vi "Test Base64 Encoder and Decoder.vi"() -> ()   [LabVIEW 2013]
uses:
  source-base64/Serializer.Base64.lvclass/Serializer.Base64.ctl
  source-base64/Base64url_CharSet.vi
  source-base64/Write charset.vi
  source-base64/Base64_CharSet.vi
  source-base64/Encode.vi
  source-base64/Serializer.Base64.lvclass
  <vilib>/LabVIEW Open Source Project/OpenSerializer/Serializer/Serializer.lvclass
panel:
  out "Decoded String":string
  out "Encoded String":string
  out "Variant 4":variant
  out "invalid type":errorcluster
  out "error out":errorcluster
  out "Variant 2":variant
  out "Variant":variant
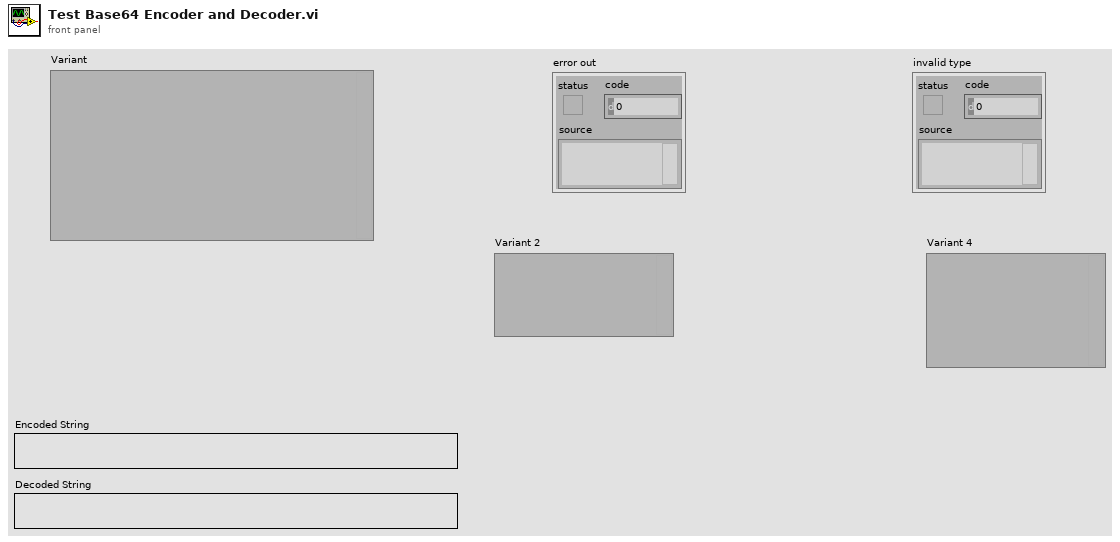
[diagram p1: front panel]
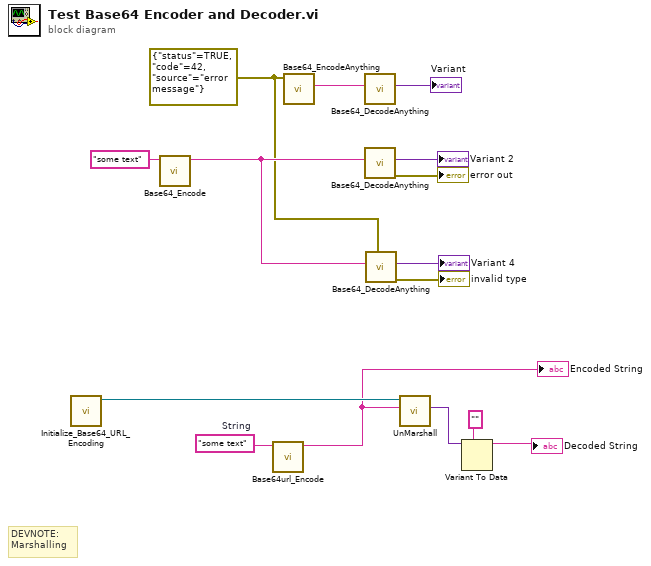
[diagram p0: block diagram]
diagram:
  w6 = "some text"  # String
  w7 = errorcluster {"status"=TRUE, "code"=42, "source"="error message"} ("error constant")
  # "DEVNOTE: \nMarshalling"
  n1 = call "Initialize_Base64_URL_Encoding.vi"() -> ("Base64 URL Encoding"=w5:refnum<class "Serializer.Base64.lvclass">)  [unwired: 11 in]
  n2 = call "Base64_Encode.vi"("String"="some text") -> ("Encoded String"=w8:string)  [unwired: 9 in, 1 out]
  n3 = call "Base64url_Encode.vi"("String"=w6) -> ("Encoded String"=w4:string)  [unwired: 9 in, 1 out]
  "Encoded String" <- w4
  n4 = call "Base64_EncodeAnything.vi"("Variant"=w7) -> ("Encoded Payload"=w14:string)  [unwired: 8 in, 2 out]
  n5 = call "Base64_DecodeAnything.vi"("Encoded Payload"=w14) -> ("Variant"=→"Variant":variant)  [unwired: 9 in, 1 out]
  n6 = call "Base64_DecodeAnything.vi"("Encoded Payload"=w8) -> ("error out"=→"error out":errorcluster, "Variant"=→"Variant 2":variant)  [unwired: 9 in]
  n7 = call "Base64_DecodeAnything.vi"("Type (Adapt)"=w7, "Encoded Payload"=w8) -> ("error out"=→"invalid type":errorcluster, "Variant"=→"Variant 4":variant)  [unwired: 8 in]
  n8 = call <vilib>:"UnMarshall.vi"("String"=w4, "Serializer in"=w5) -> ("Variant"=w3:variant)  [unwired: 7 in, 2 out]
  n9 = Variant To Data(type="", Variant=w3) -> (data=→"Decoded String":string)  [unwired: 1 in, 1 out]
